vi "Usun 0 z tablicy (SubVI).vi"(1 "all rows in":i64[][](array[numeric])) -> (0 "all rows in 2":i64[][](array[numeric]))   [LabVIEW 2013]
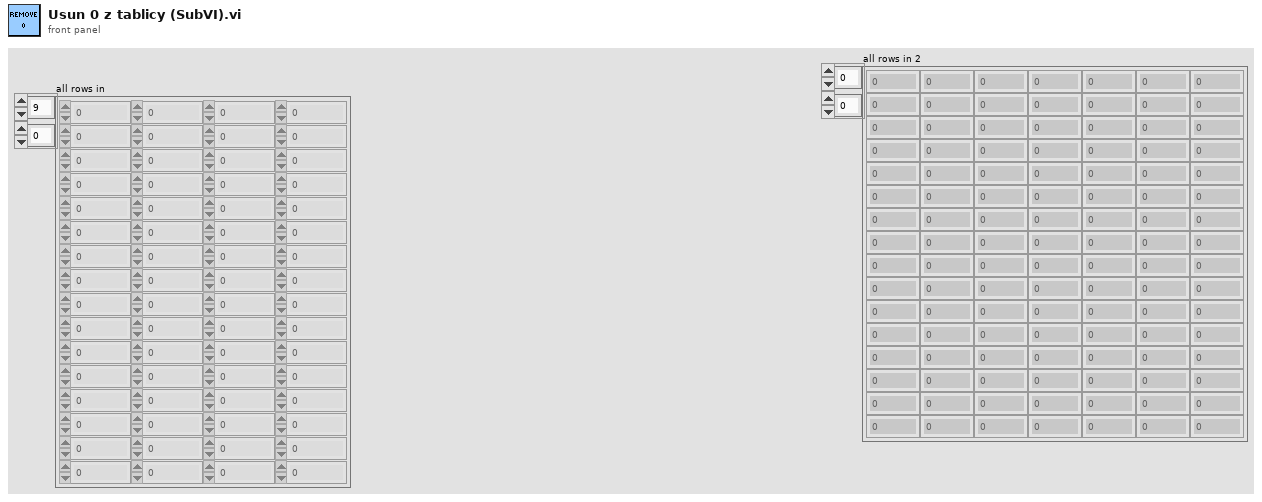
[diagram p1: front panel]
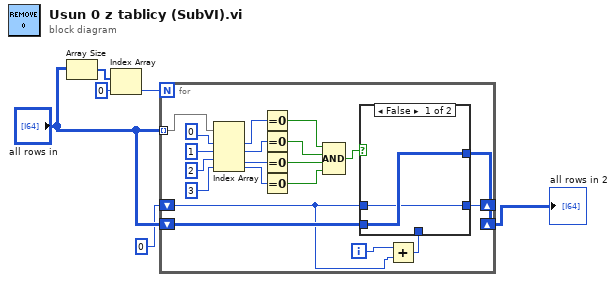
[diagram p0: block diagram]
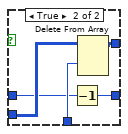
[diagram p2: hidden frame]
diagram:
  n1 = Array Size(array="all rows in") -> (size(s)=w4:i32[])
  n2 = Index Array(array=w4, index=0) -> (element=w6:i32)
  n3 = for {
    N: w6 -> [_]
    tunnel: "all rows in" -> [w13] mode=indexing
    shift-right: [w12] -> w3
    shift-left: "all rows in" -> [w11]
    shift-right: [w10] -> _
    shift-left: 0 -> [w8]
    i -> [w9]
    n4 = Index Array(array=w13, index #1=0 ("index"), index #2=1 ("index"), index #3=2 ("index"), index #4=3 ("index")) -> (element #1=w22:i64, element #2=w21:i64, element #3=w20:i64, element #4=w19:i64)
    n5 = Equal To 0?(x=w22) -> (x = 0?=w18:bool)
    n6 = Equal To 0?(x=w21) -> (x = 0?=w17:bool)
    n7 = Equal To 0?(x=w20) -> (x = 0?=w16:bool)
    n8 = Equal To 0?(x=w19) -> (x = 0?=w15:bool)
    n9 = Compound Arithmetic op=AND(w18, w17, w16, w15) -> (w14:bool)
    n10 = Add(x=w9, y=w8) -> (x+y=w7:i32)
    n11 = case shown="False" w14 {
      tunnel: w7 -> [_ w33]
      tunnel: w11 -> [w28 w32]
      tunnel: [w28 w31] -> w12
      tunnel: w8 -> [w27 w29]
      tunnel: [w27 w30] -> w10
      frame False {
      }
      frame True {
        n12 = Decrement(x=w29) -> (x-1=w30:i32)
        n13 = Delete From Array(array=w32, index (row)=w33) -> (array with subset deleted=w31:i64[][])  [unwired: 2 in, 1 out]
      }
    }
  }
  "all rows in 2" <- w3
